vi "Configure Radio Standard.vi"(0 "VISA resource name":refnum<visa-resource-name>, 1 "Band Class (0: BC0)":i32(ring) items=["BC0", "BC1"], 5 "Standard (0: None)":i32(ring) items=["None", "IS-95A", "JSTD", "IS-95C", "IS-97D", "GSM", "W3GPP", "C2000MC1", "C20001X", "NADC", "PDC", "Bluetooth", "TETRA", "WL802DOT11A", "WL802DOT11B", "WL802DOT11G", "HIPERLAN2", "DVBTLSN", "DVBTGPN", "DVBTIPN", "FCC15", "SDMBSE", "UWBINDOOR"], 7 "Enable Non-Std Measurements (F: Disable)":bool, 9 "Packet Type (0: DH1)":i32(ring) items=["DH1", "DH3", "DH5"], 11 "error in (no error)":errorcluster, 12 "Device BTS/MS (0: BTS)":i32(ring) items=["BTS", "MS"]) -> (4 "VISA resource name out":refnum<visa-resource-name>, 15 "error out":errorcluster)   [LabVIEW 2014, in "Agilent MXA Series.lvlib"]
doc: "Configures the available radio standard."
uses:
  Agilent MXA Series.lvlib
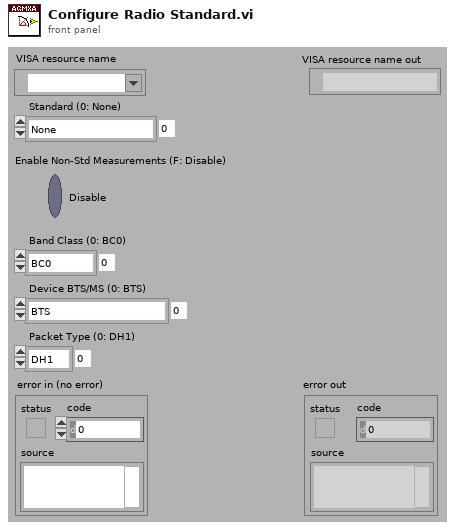
[diagram p1: front panel]
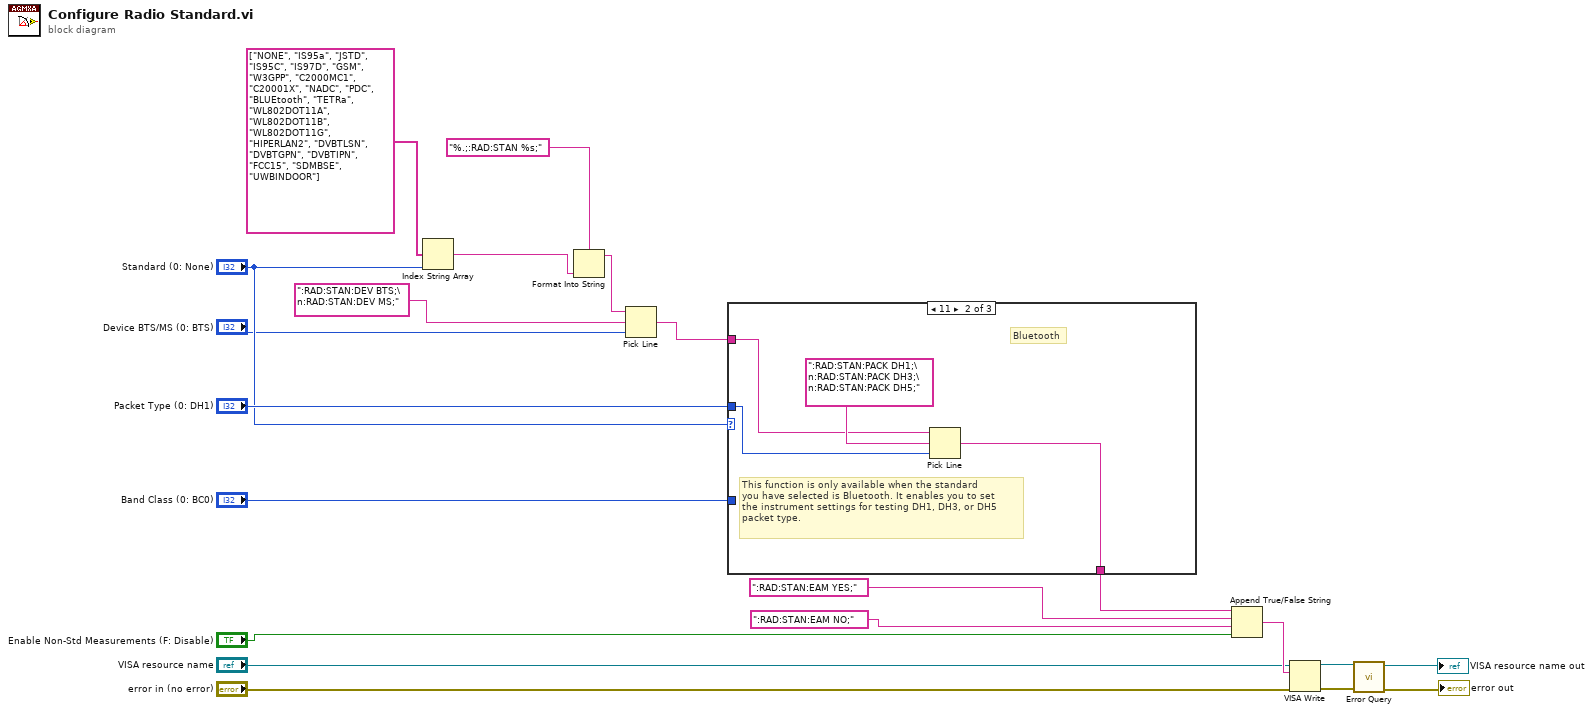
[diagram p0: block diagram]
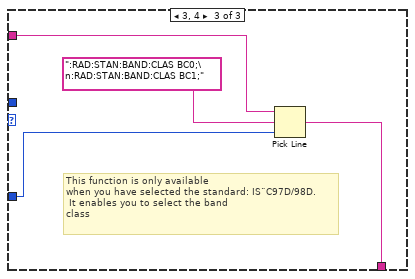
[diagram p3: hidden frame]
diagram:
  n1 = Index String Array(1:"Standard (0: None)", 2:string[] ["NONE", "IS95a", "JSTD", "IS95C", "IS97D", "GSM", "W3GPP", "C2000MC1", "C20001X", "NADC", "PDC", "BLUEtooth", "TETRa", "WL802DOT11A", "WL802DOT11B", "WL802DOT11G", "HIPERLAN2", "DVBTLSN", "DVBTGPN", "DVBTIPN", "FCC15", "SDMBSE", "UWBINDOOR"]) -> (0:w21:string)  [unwired: 1 in]
  n2 = Format Into String(format string="%.;:RAD:STAN %s;", w21) -> (resulting string=w2:string)  [unwired: 2 in, 1 out]
  n3 = Pick Line(string ("")=w2, multi-line string=":RAD:STAN:DEV BTS;\n:RAD:STAN:DEV MS;", line index="Device BTS/MS (0: BTS)") -> (output string=w1:string)
  n4 = case shown="11" "Standard (0: None)" {
    tunnel: "Packet Type (0: DH1)" -> [_ w26 _]
    tunnel: w1 -> [w22 w24 w27]
    tunnel: "Band Class (0: BC0)" -> [_ _ w30]
    tunnel: [w22 w23 w28] -> w13
    frame 0, Default {
    }
    frame 11 {
      # "This function is only available when the standard \nyou have selected is Bluetooth. It enables you to set \nthe instrument settings for testing DH1, DH3, or DH5 \npacket type."
      # "Bluetooth"
      n5 = Pick Line(string ("")=w24, multi-line string=":RAD:STAN:PACK DH1;\n:RAD:STAN:PACK DH3;\n:RAD:STAN:PACK DH5;", line index=w26) -> (output string=w23:string)
    }
    frame 3, 4 {
      # "This function is only available \nwhen you have selected the standard: IS¨C97D/98D.\n It enables you to select the band\nclass"
      n6 = Pick Line(string ("")=w27, multi-line string=":RAD:STAN:BAND:CLAS BC0;\n:RAD:STAN:BAND:CLAS BC1;", line index=w30) -> (output string=w28:string)
    }
  }
  n7 = Append True/False String(1:"Enable Non-Std Measurements (F: Disable)", 2:":RAD:STAN:EAM NO;" ("true string"), 3:":RAD:STAN:EAM YES;" ("true string"), 4:w13) -> (0:w12:string)
  n8 = VISA Write(VISA resource name="VISA resource name", write buffer=w12, error in (no error)="error in (no error)") -> (VISA resource name out=w9:refnum<visa-resource-name>, error out=w8:errorcluster)  [unwired: 1 out]
  n9 = call "Error Query.vi"("error in (no error)"=w8, "VISA resource name"=w9) -> ("error out"=→"error out":errorcluster, "VISA resource name out"=→"VISA resource name out":refnum<visa-resource-name>)  [unwired: 6 in, 2 out]
